vi "Write Snap.vi"(5 "Snap":bool, 9 "Knob in":refnum<class "Knob.lvclass">) -> (3 "Knob out":refnum<class "Knob.lvclass">)   [LabVIEW 2014, in "Knob.lvclass"]
uses:
  Knob.lvclass
  Knob.lvclass/Knob.ctl
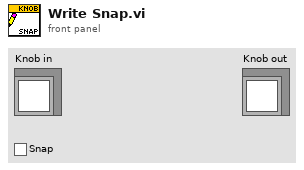
[diagram p1: front panel]
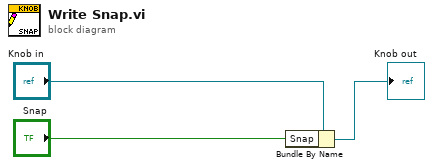
[diagram p0: block diagram]
diagram:
  n1 = Bundle By Name(cluster="Knob in", "Snap"="Snap") -> (→"Knob out":refnum<class "Knob.lvclass">)
